vi "KLB globals.vi"() -> ()   [LabVIEW 2012]
uses:
  VIs/Type Defs/KLB Settings Cluster.ctl
  VIs/Type Defs/KLB # of CPUs enum.ctl
  VIs/Type Defs/KLB compression type enum.ctl
  KLB.lvlib
panel:
  in  "KLB Settings":T1={"Logical Cores"=enum."4", "pixelSize (um)"=[1.0, 1.0, 1.0, 1.0, 1.0], "blockSize"=[96, 96, 8, 1, 1], "compressionType"=enum."BZip2", "metadata"=""} {"pixelSize (um)" min=0.01 max=10 step=0.01 format="%.2f"}
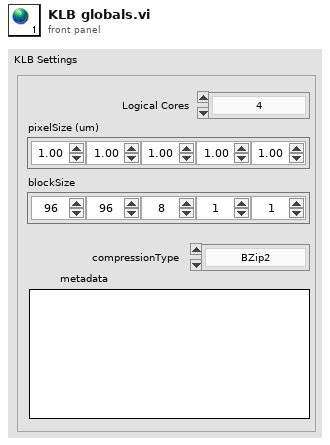
[diagram p1: front panel]
types:
  T1 = typedef "KLB.lvlib/KLB Settings Cluster.ctl" = cluster{"Logical Cores":T2, "pixelSize (um)":sgl[], "blockSize":u32[], "compressionType":T3, "metadata":string}
  T2 = typedef "KLB.lvlib/KLB # of CPUs enum.ctl" = enum16{"CPU 25%", "CPU 50%", "CPU 75%", "CPU All but 1", "1", "4", "8", "16"}
  T3 = typedef "KLB.lvlib/KLB compression type enum.ctl" = enum8{"Uncompressed", "BZip2"}
diagram:
